vi "Main.vi"() -> ()   [LabVIEW 2014]
uses:
  Lib/Formula/EnumFormula.ctl
  <vilib>/Utility/miscctls.llb/LVRowAndColumnTypeDef.ctl
  <vilib>/Utility/file.llb/Read From Spreadsheet File (string).vi
  Lib/Formula/Formula(Table).vi
  Lib/Formula/Formula(Scalar).vi
  <vilib>/Utility/file.llb/Write To Spreadsheet File (string).vi
  GlobalData/GlobalData.vi
panel:
  in  "停止":bool
  in  "タブ制御器":T1(tab)
  in  "サンプリング周期(sec)":dbl=0.002 min=1e-05 format="%#.6f"
  in  "getCh":bool
  in  "rowChNum":i32=2
  in  "rowCutNum":i32
  in  "cutRow":bool
  in  "READ":bool
  in  "rowChPos":i32=2 caption="CH名称範囲"
  in  "rowCutPos":i32 caption="ヘッダ部削除範囲"
  in  "入力データファイル":path
  in  "colCutNum":i32=2
  in  "cutCol":bool
  in  "colCutPos":i32=9 caption="不要列削除範囲"
  in  "Waveグラフ表示":bool
  in  "XYグラフ表示":bool
  in  "X軸列(1～)":i32=2
  in  "直接数値入力する":bool
  in  "B2値":dbl
  in  "追加となるCH名称":string
  in  "列追加":bool
  in  "B値":u16(ring) items=["No.", "時間HH:MM:SS.S", "M1回転rpm", "M2回転rpm", "M3回転rpm", "M1トルクN･m", "M2トルクN･m", "M3トルクN･m", "", "", "", "", "", "", "", "", "", "", "供試体温度1℃", "供試体温度2℃", "供試体温度3℃", "動力盤温度℃", "軸受温度1℃", "軸受温度2℃", "軸受温度3℃", "", "効率"]
  in  "式":T2
  in  "A値":u16(ring) items=["No.", "時間HH:MM:SS.S", "M1回転rpm", "M2回転rpm", "M3回転rpm", "M1トルクN･m", "M2トルクN･m", "M3トルクN･m", "", "", "", "", "", "", "", "", "", "", "供試体温度1℃", "供試体温度2℃", "供試体温度3℃", "動力盤温度℃", "軸受温度1℃", "軸受温度2℃", "軸受温度3℃", "", "効率"]
  in  "WRITE":bool
  in  "出力ファイル名":path
  in  "出力ファイル名（TDMS形式）":path
  in  "TDMSViewer":bool
  in  "TDMSで保存":bool
  in  "操作（0:open）":T3(ring)=enum."create or replace"
  in  "グループ名":string
  in  "新グラフ":bool
  in  "Nixedグラフ表示":bool
  in  "GraphViewer":bool
  in  "表":string[][](table)
  # "~"
  # "~"
  # "行"
  # "~"
  # "列"
  # "行"
  # "列を追加する"
  # "＝"
  # "テキスト形式でファイル保存"
  # "複数の波形データを１つのTDMSファイル形式にまとめる事が可能。"
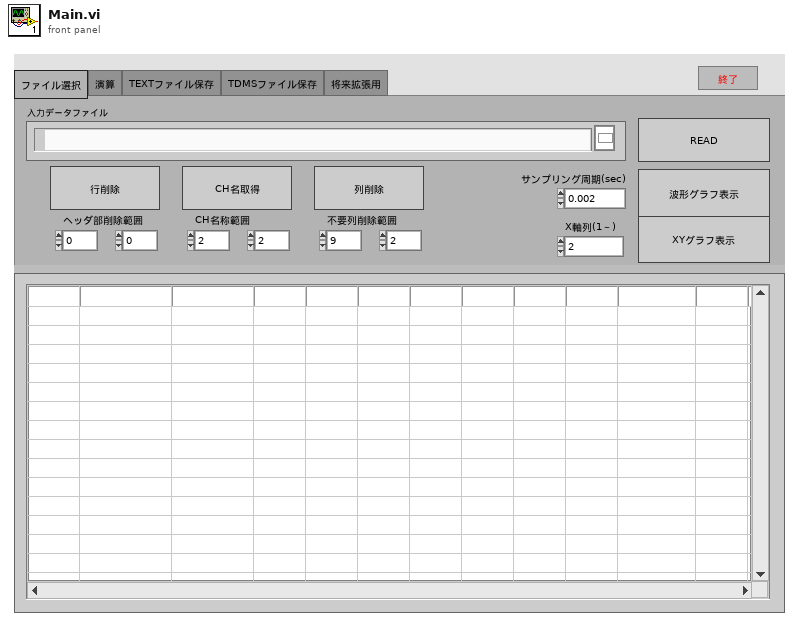
[diagram p1: front panel]
types:
  T1 = enum32{"ファイル選択", "演算", "TEXTファイル保存", "TDMSファイル保存", "将来拡張用"}
  T2 = typedef "EnumFormula.ctl" = enum16{"＋", "－", "×"}
  T3 = enum16{"open", "open or create", "create or replace", "create", "open (read-only)"}
  T4 = enum8{"Enabled", "Disabled", "Disabled and Grayed Out"}
  T5 = typedef "LVRowAndColumnTypeDef.ctl" = cluster{"Row":i32, "Column":i32}
  T6 = enum32{"Invalid", "Standard", "Closed", "Hidden", "Minimized", "Maximized"}
  T7 = typedef "LVRowAndColumnUnsignedTypeDef.ctl" = cluster{"Row":u32, "Column":u32}
  T8 = typedef "BoolSignalChangeCheck.ctl" = enum16{"OFF中", "立上り", "立下り", "ON中"}
  T9 = enum32{"Bad", "Idle", "Run top level", "Running"}
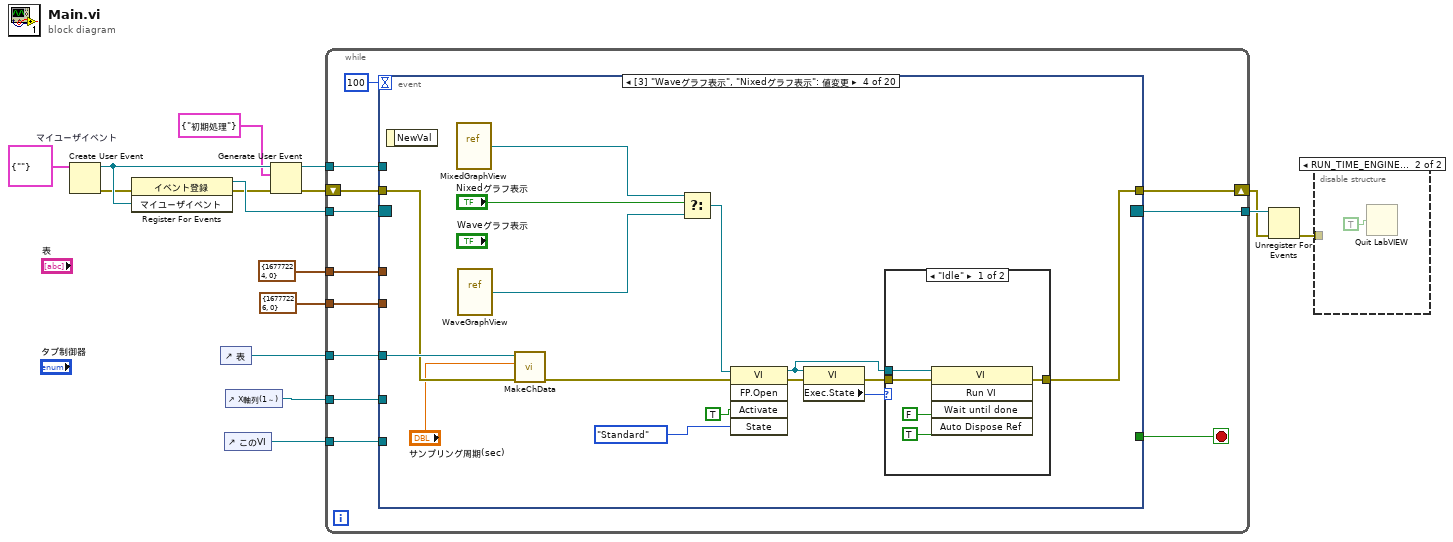
[diagram p0: block diagram]
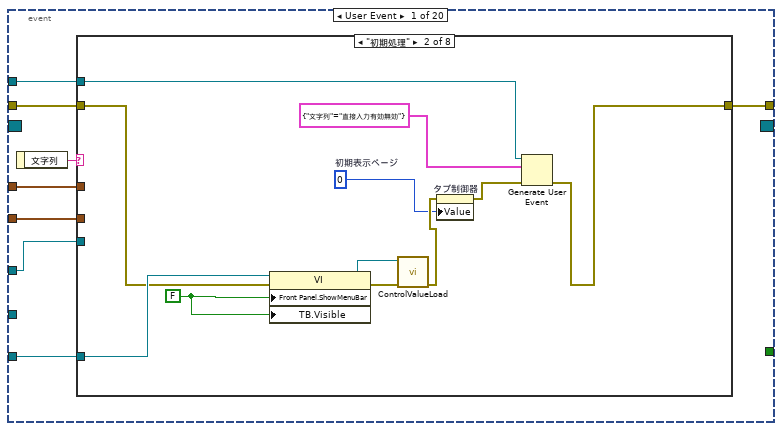
[diagram p3: hidden frame]
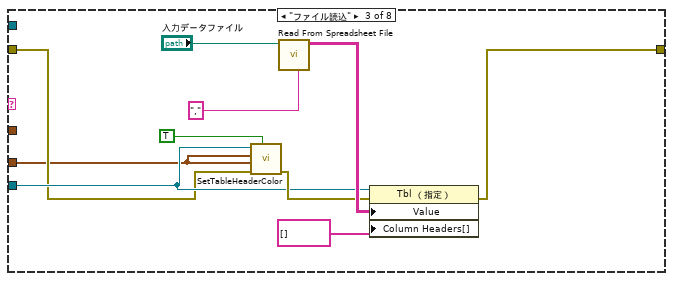
[diagram p5: hidden frame]
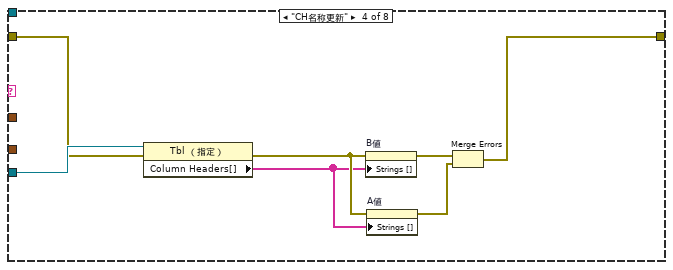
[diagram p6: hidden frame]
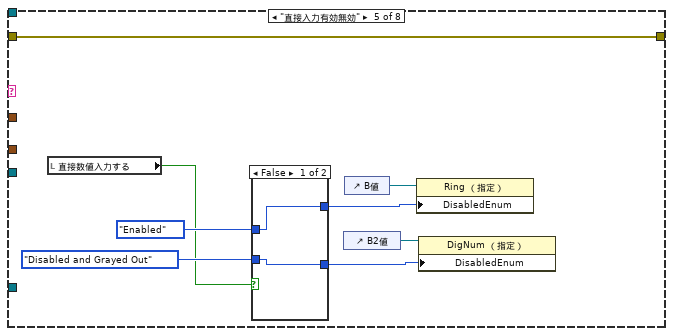
[diagram p7: hidden frame]
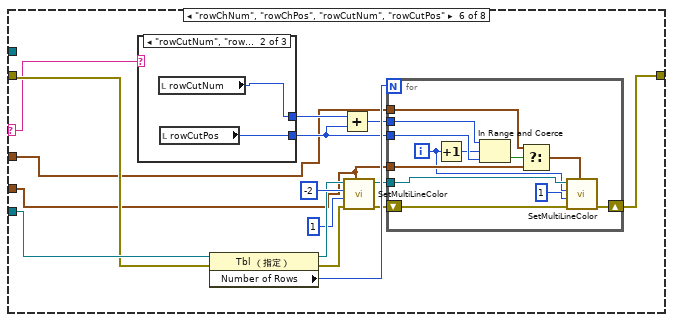
[diagram p9: hidden frame]
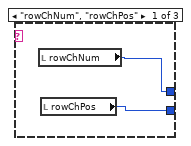
[diagram p10: hidden frame]
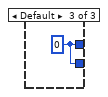
[diagram p11: hidden frame]
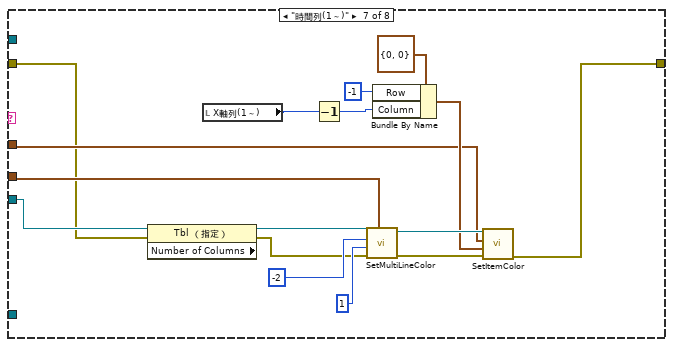
[diagram p12: hidden frame]
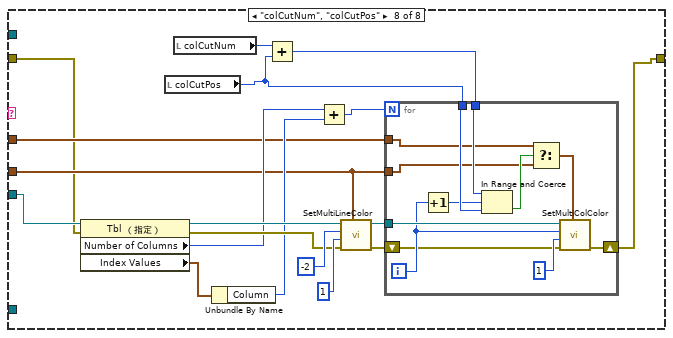
[diagram p13: hidden frame]
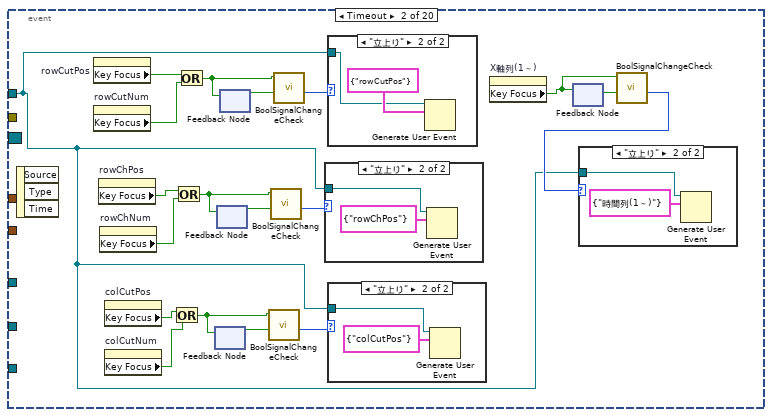
[diagram p14: hidden frame]
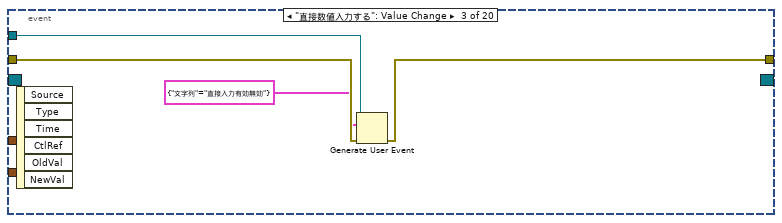
[diagram p19: hidden frame]
diagram:
  w12 = cluster{"文字列":string} {"文字列"=""}  # マイユーザイベント
  n1 = Create User Event(user event datatype=w12) -> (user event=w14:refnum<user-event>, error out=w5:errorcluster)  [unwired: 1 in]
  n2 = register-events(error in=w5, w14) -> (reference out=w16:refnum<event-registration>, error out=w4:errorcluster)  [unwired: 1 in]
  n3 = control-ref of="表"() -> (w10:refnum<vi>)
  n4 = control-ref of="このVI"() -> (w6:refnum<vi>)
  n5 = control-ref of="X軸列(1～)"() -> (w7:refnum<vi>)
  n6 = Generate User Event(user event=w14, event data cluster=cluster{"文字列":string} {"文字列"="初期処理"} ("イベントデータ"), error in=w4) -> (user event out=w13:refnum<user-event>, error out=w3:errorcluster)  [unwired: 1 in]
  n7 = while {
    tunnel: w16 -> [w27]
    tunnel: w13 -> [w26]
    tunnel: [w25] -> w15
    tunnel: w10 -> [w24]
    tunnel: cluster{"背景色":u32, "文字色":u32} {"背景色"=16777226, "文字色"=0} ("色指定") -> [w23]
    tunnel: cluster{"背景色":u32, "文字色":u32} {"背景色"=16777224, "文字色"=0} ("色指定") -> [w22]
    tunnel: w7 -> [w21]
    tunnel: w6 -> [w20]
    shift-right: [w18] -> w1
    shift-left: w3 -> [w19]
    stop <- w28 stop-if-true
    n8 = event shown="[3] \"Waveグラフ表示\", \"Nixedグラフ表示\": 値変更" {
      selector: w27 -> [_ _ _ _ _ _ _ _ _ _ _ _ _ _ _ _ _ _ _ _]
      dyn-events: [_ _ _ _ _ _ _ _ _ _ _ _ _ _ _ _ _ _ _ _] -> w25
      timeout: 100 -> [_ _ _ _ _ _ _ _ _ _ _ _ _ _ _ _ _ _ _ _]
      tunnel: [_ _ _ _ _ _ _ _ _ _ _ _ _ _ _ _ _ _ _ "停止"] -> w28
      tunnel: w26 -> [w35 w157 w184 _ _ _ w235 _ _ _ _ w315 w319 w323 w335 w336 _ w361 w386 _]
      tunnel: w24 -> [w34 _ _ w192 w211 w218 w232 w258 _ w278 w300 _ _ _ _ _ w343 w376 w383 w412]
      tunnel: w23 -> [w30 _ _ _ _ _ _ _ _ _ _ _ _ _ _ _ w356 w370 w389 w410]
      tunnel: w22 -> [w29 _ _ _ _ _ _ _ _ _ _ _ _ _ _ _ _ _ _ _]
      tunnel: w21 -> [_ _ _ _ _ w219 _ _ _ _ _ _ _ _ _ _ _ _ _ _]
      tunnel: w20 -> [w33 _ _ _ _ _ _ _ _ _ _ _ _ _ _ _ _ _ _ w403]
      tunnel: w19 -> [w32 _ w187 w191 w213 w217 w226 w255 w271 w277 w298 w316 w318 w327 w334 w342 w344 w358 w385 w406]
      tunnel: [w31 _ w186 w189 w212 w215 w223 w253 w270 _ w297 w313 w317 w321 w333 w341 w345 w359 w384 w400] -> w18
      event User Event {
        n9 = event-data() -> ("文字列"=w36:string)  [unwired: 1 in]
        n10 = case shown="\"初期処理\"" w36 {
          selector: w36 -> [_ _ _ _ _ w81 _ _]
          tunnel: w35 -> [_ w42 _ _ _ _ _ _]
          tunnel: w34 -> [_ _ w52 w65 _ w83 w113 w129]
          tunnel: w33 -> [_ w47 _ _ _ _ _ _]
          tunnel: w32 -> [w37 w45 w51 w64 w67 w82 w112 w127]
          tunnel: [w37 w41 w50 w60 w67 w80 w111 w128] -> w31
          tunnel: w30 -> [_ _ w49 _ _ w78 w114 w130]
          tunnel: w29 -> [_ _ _ _ _ w79 w115 w131]
          frame Default {
          }
          frame "初期処理" {
            w38 = u32 0  # 初期表示ページ
            w48 = FALSE
            n11 = property class="VI"(reference=w47, error in=w45, "Front Panel.ShowMenuBar"=w48, "TB.Visible"=w48) -> (reference out=w46:refnum<vi>, error out=w44:errorcluster)
            n12 = call "ControlValueLoad.vi"("err(in)"=w44, "VI refnum"=w46) -> ("err(out)"=w39:errorcluster)  [unwired: 9 in]
            n13 = property on="タブ制御器" class="TabCtl （指定）"(error in=w39, "Value"=w38) -> (error out=w40:errorcluster)  [unwired: 1 in, 1 out]
            n14 = Generate User Event(user event=w42, event data cluster=cluster{"文字列":string} {"文字列"="直接入力有効無効"} ("イベントデータ"), error in=w40) -> (error out=w41:errorcluster)  [unwired: 1 in, 1 out]
          }
          frame "ファイル読込" {
            n15 = call "SetTableHeaderColor.vi"("セル塗?(F)"=TRUE, "エラー入力(エラーなし)"=w51, "セル色指定"=w49, "ヘッダー色指定"=w49, "Tbl refnum"=w52) -> ("エラー出力"=w53:errorcluster)  [unwired: 6 in]
            n16 = call-poly <vilib>:"Read From Spreadsheet File.vi"("delimiter (\\t)"="," ("delimiter (\\t)"), "file path (dialog if empty)"="入力データファイル") -> ("all rows"=w55:string[][])  [unwired: 5 in, 4 out]
            n17 = property class="Tbl （指定）"(reference=w52, error in=w53, "Value"=w55, "Column Headers[]"=string[] [] ("行ヘッダ文字列[]")) -> (error out=w50:errorcluster)  [unwired: 1 out]
          }
          frame "CH名称更新" {
            n18 = property class="Tbl （指定）"(reference=w65, error in=w64) -> (error out=w63:errorcluster, "Column Headers[]"=w59:string[])  [unwired: 1 out]
            n19 = property on="B値" class="Ring （指定）"(error in=w63, "Strings []"=w59) -> (error out=w62:errorcluster)  [unwired: 1 in, 1 out]
            n20 = property on="A値" class="Ring （指定）"(error in=w63, "Strings []"=w59) -> (error out=w61:errorcluster)  [unwired: 1 in, 1 out]
            n21 = Merge Errors(w62, w61) -> (w60:errorcluster)
          }
          frame "直接入力有効無効" {
            n22 = local read "直接数値入力する"() -> (w66:bool)
            n23 = case shown="FALSE" w66 {
              tunnel: [w75 w77] -> w71
              tunnel: T4."Enabled" ("無効") -> [w74 w77]
              tunnel: [w74 w76] -> w69
              tunnel: T4."Disabled and Grayed Out" ("無効") -> [w75 w76]
              frame False {
              }
              frame True {
              }
            }
            n24 = control-ref of="B2値"() -> (w72:refnum<vi>)
            n25 = control-ref of="B値"() -> (w73:refnum<vi>)
            n26 = property class="Ring （指定）"(reference=w73, "DisabledEnum"=w69) -> ()  [unwired: 1 in, 2 out]
            n27 = property class="DigNum （指定）"(reference=w72, "DisabledEnum"=w71) -> ()  [unwired: 1 in, 2 out]
          }
          frame "rowChNum", "rowChPos", "rowCutNum", "rowCutPos" {
            n28 = case shown="\"rowCutNum\", \"rowCutPos\"" w81 {
              tunnel: [w95 w97 w98] -> w90
              tunnel: [w94 w96 w98] -> w92
              frame "rowChNum", "rowChPos" {
                n29 = local read "rowChNum"() -> (w95:i32)
                n30 = local read "rowChPos"() -> (w94:i32)
              }
              frame "rowCutNum", "rowCutPos" {
                n31 = local read "rowCutNum"() -> (w97:i32)
                n32 = local read "rowCutPos"() -> (w96:i32)
              }
              frame Default {
                w98 = 0
              }
            }
            n33 = property class="Tbl （指定）"(reference=w83, error in=w82) -> (reference out=w87:refnum<vi>, error out=w85:errorcluster, "Number of Rows"=w93:u32)
            n34 = Add(x=w90, y=w92) -> (x+y=w91:i32)
            n35 = call "SetMultiLineColor.vi"("色指定"=w78, "Error In"=w85, "長さ"=1, "開始行"=-2, "Tbl refnum"=w87) -> ("Error Out"=w84:errorcluster, "Tbl refnum出力"=w88:refnum<vi>)  [unwired: 5 in]
            n36 = for {
              N: w93 -> [_]
              tunnel: w91 -> [w110]
              tunnel: w92 -> [w109]
              tunnel: w79 -> [w107]
              tunnel: w78 -> [w106]
              tunnel: w88 -> [w104]
              shift-right: [w99] -> w80
              shift-left: w84 -> [w100]
              i -> [w103]
              n37 = Increment(x=w103) -> (x+1=w101:i32)
              n38 = In Range and Coerce(upper limit=w110, x=w101, lower limit=w109) -> (In Range?=w108:bool)  [unwired: 1 out]
              n39 = Select(t=w107, s=w108, f=w106) -> (s? t:f=w105:cluster{"背景色":u32, "文字色":u32})
              n40 = call "SetMultiLineColor.vi"("色指定"=w105, "Error In"=w100, "長さ"=1, "開始行"=w103, "Tbl refnum"=w104) -> ("Error Out"=w99:errorcluster)  [unwired: 5 in, 1 out]
            }
          }
          frame "時間列(1～)" {
            n41 = property class="Tbl （指定）" props=["Number of Columns"](reference=w113, error in=w112) -> (reference out=w126:refnum<vi>, error out=w123:errorcluster)  [unwired: 1 out]
            n42 = local read "X軸列(1～)"() -> (w116:i32)
            n43 = Decrement(x=w116) -> (x-1=w117:i32)
            n44 = call "SetMultiLineColor.vi"("色指定"=w114, "Error In"=w123, "長さ"=1, "開始行"=-2, "Tbl refnum"=w126) -> ("Error Out"=w119:errorcluster, "Tbl refnum出力"=w120:refnum<vi>)  [unwired: 5 in]
            n45 = Bundle By Name(cluster=T5 {"Row"=0, "Column"=0} ("行列指定"), "Row"=-1, "Column"=w117) -> (w118:T5)
            n46 = call "SetItemColor.vi"("エラー入力(エラーなし)"=w119, "行列指定"=w118, "色指定"=w115, "Tbl refnum"=w120) -> ("エラー出力"=w111:errorcluster)  [unwired: 7 in]
          }
          frame "colCutNum", "colCutPos" {
            n47 = property class="Tbl （指定）"(reference=w129, error in=w127) -> (reference out=w142:refnum<vi>, error out=w139:errorcluster, "Number of Columns"=w135:u32, "Index Values"=w137:T7)
            n48 = local read "colCutPos"() -> (w132:i32)
            n49 = local read "colCutNum"() -> (w133:i32)
            n50 = Unbundle By Name(w137) -> ("Column"=w136:u32)
            n51 = Add(x=w133, y=w132) -> (x+y=w144:i32)
            n52 = Add(x=w135, y=w136) -> (x+y=w134:u32)
            n53 = call "SetMultiLineColor.vi"("色指定"=w130, "Error In"=w139, "長さ"=1, "開始行"=-2, "Tbl refnum"=w142) -> ("Error Out"=w138:errorcluster, "Tbl refnum出力"=w141:refnum<vi>)  [unwired: 5 in]
            n54 = for {
              N: w134 -> [_]
              tunnel: w144 -> [w156]
              tunnel: w132 -> [w155]
              tunnel: w131 -> [w153]
              tunnel: w130 -> [w152]
              tunnel: w141 -> [w150]
              shift-right: [w145] -> w128
              shift-left: w138 -> [w146]
              i -> [w149]
              n55 = Increment(x=w149) -> (x+1=w147:i32)
              n56 = In Range and Coerce(upper limit=w156, x=w147, lower limit=w155) -> (In Range?=w154:bool)  [unwired: 1 out]
              n57 = Select(t=w153, s=w154, f=w152) -> (s? t:f=w151:cluster{"背景色":u32, "文字色":u32})
              n58 = call "SetMultiColColor.vi"("色指定"=w151, "Error In"=w146, "長さ"=1, "開始列"=w149, "Tbl refnum"=w150) -> ("Error Out"=w145:errorcluster)  [unwired: 5 in, 1 out]
            }
          }
        }
      }
      event Timeout {
        n59 = event-data() -> ()  [unwired: 1 in, 3 out]
        n60 = property on="rowCutPos" class="DigNum （指定）"() -> ("Key Focus"=w175:bool)  [unwired: 2 in, 2 out]
        n61 = property on="rowCutNum" class="DigNum （指定）"() -> ("Key Focus"=w174:bool)  [unwired: 2 in, 2 out]
        n62 = property on="rowChPos" class="DigNum （指定）"() -> ("Key Focus"=w167:bool)  [unwired: 2 in, 2 out]
        n63 = property on="rowChNum" class="DigNum （指定）"() -> ("Key Focus"=w166:bool)  [unwired: 2 in, 2 out]
        n64 = property on="colCutPos" class="DigNum （指定）"() -> ("Key Focus"=w163:bool)  [unwired: 2 in, 2 out]
        n65 = property on="colCutNum" class="DigNum （指定）"() -> ("Key Focus"=w162:bool)  [unwired: 2 in, 2 out]
        n66 = Or(x=w163, y=w162) -> (x .or. y?=w165:bool)
        n67 = Or(x=w167, y=w166) -> (x .or. y?=w168:bool)
        n68 = Or(x=w175, y=w174) -> (x .or. y?=w173:bool)
        n69 = feedback #1() -> (w164:bool)  [unwired: 1 in]
        n70 = feedback-in #1(w165) -> ()
        n71 = feedback #2() -> (w169:bool)  [unwired: 1 in]
        n72 = feedback-in #2(w168) -> ()
        n73 = feedback-in #3(w173) -> ()
        n74 = feedback #3() -> (w172:bool)  [unwired: 1 in]
        n75 = call "BoolSignalChangeCheck.vi"("前回値"=w164, "今回値"=w165) -> ("判定"=w161:T8)  [unwired: 9 in]
        n76 = call "BoolSignalChangeCheck.vi"("前回値"=w169, "今回値"=w168) -> ("判定"=w170:T8)  [unwired: 9 in]
        n77 = call "BoolSignalChangeCheck.vi"("前回値"=w172, "今回値"=w173) -> ("判定"=w171:T8)  [unwired: 9 in]
        n78 = case shown="\"立上り\"" w170 {
          tunnel: w157 -> [_ w180]
          frame "OFF中", Default {
          }
          frame "立上り" {
            n79 = Generate User Event(user event=w180, event data cluster=cluster{"文字列":string} {"文字列"="rowChPos"} ("イベントデータ")) -> ()  [unwired: 2 in, 2 out]
          }
        }
        n80 = case shown="\"立上り\"" w171 {
          tunnel: w157 -> [_ w182]
          frame "OFF中", Default {
          }
          frame "立上り" {
            n81 = Generate User Event(user event=w182, event data cluster=cluster{"文字列":string} {"文字列"="rowCutPos"} ("イベントデータ")) -> ()  [unwired: 2 in, 2 out]
          }
        }
        n82 = case shown="\"立上り\"" w161 {
          tunnel: w157 -> [_ w178]
          frame "OFF中", Default {
          }
          frame "立上り" {
            n83 = Generate User Event(user event=w178, event data cluster=cluster{"文字列":string} {"文字列"="colCutPos"} ("イベントデータ")) -> ()  [unwired: 2 in, 2 out]
          }
        }
        n84 = property on="X軸列(1～)" class="DigNum （指定）"() -> ("Key Focus"=w160:bool)  [unwired: 2 in, 2 out]
        n85 = feedback #4() -> (w159:bool)  [unwired: 1 in]
        n86 = feedback-in #4(w160) -> ()
        n87 = call "BoolSignalChangeCheck.vi"("前回値"=w159, "今回値"=w160) -> ("判定"=w158:T8)  [unwired: 9 in]
        n88 = case shown="\"立上り\"" w158 {
          tunnel: w157 -> [_ w176]
          frame "OFF中", Default {
          }
          frame "立上り" {
            n89 = Generate User Event(user event=w176, event data cluster=cluster{"文字列":string} {"文字列"="時間列(1～)"} ("イベントデータ")) -> ()  [unwired: 2 in, 2 out]
          }
        }
      }
      event "直接数値入力する": Value Change {
        n90 = event-data() -> ()  [unwired: 1 in, 6 out]
        n91 = Generate User Event(user event=w184, event data cluster=cluster{"文字列":string} {"文字列"="直接入力有効無効"} ("イベントデータ"), error in=w187) -> (error out=w186:errorcluster)  [unwired: 1 in, 1 out]
      }
      event "Waveグラフ表示", "Nixedグラフ表示": Value Change {
        n92 = event-data() -> ()  [unwired: 1 in, 1 out]
        n93 = vi-ref "MixedGraphView.vi"() -> (w196:refnum<vi>)
        n94 = vi-ref "WaveGraphView.vi"() -> (w195:refnum<vi>)
        n95 = call "MakeChData.vi"("error in (no error)"=w191, "サンプリング周期(sec)"="サンプリング周期(sec)", "表 ref"=w192) -> ("error out"=w193:errorcluster)  [unwired: 8 in]
        n96 = Select(t=w196, s="Nixedグラフ表示", f=w195) -> (s? t:f=w194:refnum<vi>)
        n97 = invoke class="VI" method="FP.Open"(reference=w194, error in=w193, "Activate"=TRUE ("アクティブ化?"), "State"=T6."Standard" ("状態")) -> (reference out=w200:refnum<vi>, error out=w199:errorcluster)  [unwired: 1 in, 3 out]
        n98 = property class="VI"(reference=w200, error in=w199) -> (error out=w190:errorcluster, "Exec.State"=w198:T9)  [unwired: 1 out]
        n99 = case shown="\"Idle\"" w198 {
          tunnel: w200 -> [w205 _]
          tunnel: w190 -> [w204 w208]
          tunnel: [w203 w208] -> w189
          frame "Idle" {
            n100 = invoke class="VI" method="Run VI"(reference=w205, error in=w204, "Wait until done"=FALSE ("終了まで待機"), "Auto Dispose Ref"=TRUE ("リファレンスを自動破棄")) -> (error out=w203:errorcluster)  [unwired: 1 in, 4 out]
          }
          frame Default {
          }
        }
      }
      event "新グラフ": Value Change {
        n101 = event-data() -> ()  [unwired: 1 in, 1 out]
        n102 = vi-ref "GraphView.vi"() -> (w210:refnum<vi>)
        n103 = local read "サンプリング周期(sec)"() -> (w209:dbl)
        n104 = call "MakeChData.vi"("error in (no error)"=w213, "サンプリング周期(sec)"=w209, "表 ref"=w211) -> ("error out"=w214:errorcluster)  [unwired: 8 in]
        n105 = call "FormPopup.vi"("エラー入力（エラーなし）"=w214, "VI入力"=w210) -> ("エラー出力"=w212:errorcluster)  [unwired: 9 in]
      }
      event "XYグラフ表示": Value Change {
        n106 = event-data() -> ()  [unwired: 1 in, 1 out]
        n107 = call "MakeXyData.vi"("error in (no error)"=w217, "時間列(1～) ref"=w219, "表 ref"=w218) -> ("error out"=w216:errorcluster)  [unwired: 8 in]
        n108 = vi-ref "XYGraphView.vi"() -> (w220:refnum<vi>)
        n109 = call "FormPopup.vi"("エラー入力（エラーなし）"=w216, "VI入力"=w220) -> ("エラー出力"=w215:errorcluster)  [unwired: 9 in]
      }
      event "列追加": Value Change {
        n110 = event-data() -> ()  [unwired: 1 in, 1 out]
        n111 = property class="Tbl （指定）"(reference=w232, error in=w226) -> (reference out=w230:refnum<vi>, error out=w225:errorcluster, "Value"=w222:string[][])
        n112 = Transpose 2D Array(2D array=w222) -> (transposed array=w221:string[][])
        n113 = case shown="TRUE" "直接数値入力する" {
          tunnel: "A値" -> [w244 w250]
          tunnel: "B値" -> [w243 _]
          tunnel: [w241 w252] -> w236
          tunnel: "B2値" -> [_ w249]
          tunnel: "式" -> [w242 w248]
          tunnel: w221 -> [w245 w251]
          tunnel: w225 -> [w240 w247]
          tunnel: [w239 w246] -> w224
          frame False {
            n114 = call-poly "Formula.vi"("式"=w242, "error in (no error)"=w240, "B値(列位置 0～)"=w243, "A値(列位置 0～)"=w244, "元データ(2D)"=w245) -> ("error out"=w239:errorcluster, "結果データ(1D)"=w241:dbl[])  [unwired: 5 in]
          }
          frame True {
            n115 = call-poly "Formula.vi"("式"=w248, "error in (no error)"=w247, "B(値)"=w249, "A(列位置 0～)"=w250, "元データ(2D)"=w251) -> ("error out"=w246:errorcluster, "結果データ(1D)"=w252:dbl[])  [unwired: 5 in]
          }
        }
        n116 = call "AddColData.vi"("エラー入力（エラーなし）"=w224, "名称"="追加となるCH名称", "配列"=w236, "Table入力"=w230) -> ("エラー出力"=w231:errorcluster)  [unwired: 7 in]
        n117 = Generate User Event(user event=w235, event data cluster=cluster{"文字列":string} {"文字列"="Ch名称更新"} ("イベントデータ"), error in=w231) -> (error out=w223:errorcluster)  [unwired: 1 in, 1 out]
      }
      event "WRITE": Value Change {
        n118 = event-data() -> ()  [unwired: 1 in, 1 out]
        n119 = property class="Tbl （指定）"(reference=w258, error in=w255) -> (error out=w254:errorcluster, "Column Headers[]"=w257:string[], "Value"=w256:string[][])  [unwired: 1 out]
        n120 = Build Array (concatenate)(w257, w256) -> (w259:string[][])
        n121 = call <vilib>:"Check if File or Folder Exists.vi"("error in (no error)"=w254, "path"="出力ファイル名") -> ("error out"=w253:errorcluster, "file or folder exists?"=w262:bool, "dup path"=w261:path)  [unwired: 7 in]
        n122 = case shown="TRUE" w262 {
          tunnel: [TRUE w268] -> w260
          frame False {
          }
          frame True {
            n123 = Two Button Dialog(message="上書きします。\n宜しいですか？" ("メッセージ")) -> (T button?=w268:bool)  [unwired: 2 in]
          }
        }
        n124 = case shown="TRUE" w260 {
          tunnel: w261 -> [_ w266]
          tunnel: w259 -> [_ w264]
          frame False {
          }
          frame True {
            n125 = call-poly <vilib>:"Write To Spreadsheet File.vi"("delimiter (\\t)"="," ("delimiter (\\t)"), "2D data"=w264, "file path (dialog if empty)"=w266) -> ()  [unwired: 5 in, 1 out]
          }
        }
      }
      event "TDMSViewer": Value Change {
        n126 = event-data() -> ()  [unwired: 1 in, 1 out]
        n127 = local read "出力ファイル名（TDMS形式）"() -> (w272:path)
        n128 = call <vilib>:"TDMS - File Viewer.vi"("error in (no error)"=w271, "file path"=w272) -> ("error out"=w270:errorcluster)  [unwired: 4 in, 1 out]
      }
      event "GraphViewer": Value Change {
        n129 = event-data() -> ()  [unwired: 1 in, 1 out]
        n130 = local read "サンプリング周期(sec)"() -> (w273:dbl)
        n131 = call "MakeChData.vi"("error in (no error)"=w277, "サンプリング周期(sec)"=w273, "表 ref"=w278) -> ("error out"=w276:errorcluster)  [unwired: 8 in]
        n132 = flat-sequence {
          tunnel: w276 -> [_]
          tunnel: [w283] -> w275
          tunnel: [w282] -> w274
          frame #0 {
            n133 = property on="入力データファイル" class="Path"() -> ("Text.Text"=w281:string)  [unwired: 2 in, 2 out]
            n134 = String To Path(string=w281) -> (path=w280:path)
            n135 = call <vilib>:"Application Directory.vi"() -> ("Application Directory"=w287:path)
            n136 = call <vilib>:"Get File Extension.vi"("file"=w280) -> ("filename without extension"=w279:string)  [unwired: 7 in, 3 out]
            n137 = Build Path(base path=w287, name or relative path="WaveDisp V2.tdms" ("名前または相対パス")) -> (appended path=w285:path)
            n138 = global read "GlobalData.vi" "ChName"() -> (w294:string[])
            n139 = global read "GlobalData.vi" "ChData"() -> (w293:waveform(dbl)[])
            n140 = TDMS Open(10:T3."create or replace" ("操作（0:open）"), 11:w285) -> (0:w292:errorcluster, 3:w295:refnum<k34>)  [unwired: 5 in]
            n141 = TDMS Write(0:w295, 5:w279, 7:w294, 9:w293, 11:w292) -> (4:w290:refnum<k34>, 15:w291:errorcluster)  [unwired: 1 in, 2 out]
            n142 = TDMS Flush(4:w291, 7:w290) -> (0:w289:errorcluster, 3:w288:refnum<k34>)
            n143 = TDMS Close(8:w289, 11:w288) -> (0:w283:errorcluster, 3:w282:path)
          }
        }
        n144 = call <vilib>:"TDMS - File Viewer.vi"("error in (no error)"=w275, "file path"=w274) -> ()  [unwired: 4 in, 2 out]
      }
      event "TDMSで保存": Value Change {
        n145 = event-data() -> ()  [unwired: 1 in, 1 out]
        n146 = local read "サンプリング周期(sec)"() -> (w296:dbl)
        n147 = call "MakeChData.vi"("error in (no error)"=w298, "サンプリング周期(sec)"=w296, "表 ref"=w300) -> ("error out"=w299:errorcluster)  [unwired: 8 in]
        n148 = flat-sequence {
          tunnel: w299 -> [w301]
          tunnel: [w301] -> w297
          frame #0 {
            n149 = global read "GlobalData.vi" "ChName"() -> (w308:string[])
            n150 = global read "GlobalData.vi" "ChData"() -> (w307:waveform(dbl)[])
            n151 = TDMS Open(10:"操作（0:open）", 11:"出力ファイル名（TDMS形式）") -> (0:w306:errorcluster, 3:w312:refnum<k34>)  [unwired: 5 in]
            n152 = TDMS Write(0:w312, 5:"グループ名", 7:w308, 9:w307, 11:w306) -> (4:w304:refnum<k34>, 15:w305:errorcluster)  [unwired: 1 in, 2 out]
            n153 = TDMS Flush(4:w305, 7:w304) -> (0:w303:errorcluster, 3:w302:refnum<k34>)
            n154 = TDMS Close(8:w303, 11:w302) -> ()  [unwired: 2 out]
          }
        }
      }
      event "READ": Value Change {
        n155 = event-data() -> ()  [unwired: 1 in, 1 out]
        n156 = Generate User Event(user event=w315, event data cluster=cluster{"文字列":string} {"文字列"="ファイル読込"} ("イベントデータ"), error in=w316) -> (error out=w313:errorcluster)  [unwired: 1 in, 1 out]
      }
      event "入力データファイル": Value Change {
        n157 = event-data() -> ()  [unwired: 1 in, 1 out]
        n158 = Generate User Event(user event=w319, event data cluster=cluster{"文字列":string} {"文字列"="ファイル読込"} ("イベントデータ"), error in=w318) -> (error out=w317:errorcluster)  [unwired: 1 in, 1 out]
      }
      event "rowCutPos", "rowCutNum", "rowChNum", "rowChPos": Value Change {
        n159 = event-data() -> ("CtlRef"=w328:refnum<vi>)  [unwired: 1 in]
        n160 = property class="DigNum （指定）"(reference=w328, error in=w327) -> (error out=w322:errorcluster, "Label.Text"=w325:string)  [unwired: 1 out]
        n161 = Bundle By Name(cluster=cluster{"文字列":string} {"文字列"="(項目名)"} ("イベントデータ"), "文字列"=w325) -> (w324:cluster{"文字列":string})
        n162 = Generate User Event(user event=w323, event data cluster=w324, error in=w322) -> (error out=w321:errorcluster)  [unwired: 1 in, 1 out]
      }
      event "X軸列(1～)": Value Change {
        n163 = event-data() -> ("CtlRef"=w332:refnum<vi>)  [unwired: 1 in]
        n164 = property class="DigNum （指定）"(reference=w332) -> ("Label.Text"=w330:string)  [unwired: 1 in, 2 out]
        n165 = Bundle By Name(cluster=cluster{"文字列":string} {"文字列"="(項目名)"} ("イベントデータ"), "文字列"=w330) -> (w329:cluster{"文字列":string})
        n166 = Generate User Event(user event=w335, event data cluster=w329, error in=w334) -> (error out=w333:errorcluster)  [unwired: 1 in, 1 out]
      }
      event "colCutPos", "colCutNum": Value Change {
        n167 = event-data() -> ("CtlRef"=w340:refnum<vi>)  [unwired: 1 in]
        n168 = property class="DigNum （指定）"(reference=w340) -> ("Label.Text"=w338:string)  [unwired: 1 in, 2 out]
        n169 = Bundle By Name(cluster=cluster{"文字列":string} {"文字列"="(項目名)"} ("イベントデータ"), "文字列"=w338) -> (w337:cluster{"文字列":string})
        n170 = Generate User Event(user event=w336, event data cluster=w337, error in=w342) -> (error out=w341:errorcluster)  [unwired: 1 in, 1 out]
      }
      event "cutRow": Value Change {
        n171 = event-data() -> ()  [unwired: 1 in, 1 out]
        n172 = property class="Tbl （指定）"(reference=w343, error in=w344) -> (reference out=w351:refnum<vi>, error out=w350:errorcluster, "Value"=w357:string[][])
        n173 = local read "rowCutNum"() -> (w348:i32)
        n174 = local read "rowCutPos"() -> (w349:i32)
        n175 = Decrement(x=w349) -> (x-1=w346:i32)
        n176 = Delete From Array(array=w357, length=w348, index (row)=w346) -> (array with subset deleted=w347:string[][])  [unwired: 1 in, 1 out]
        n177 = property class="Tbl （指定）"(reference=w351, error in=w350, "Value"=w347) -> (reference out=w355:refnum<vi>, error out=w352:errorcluster, "Number of Rows"=w353:u32)
        n178 = call "SetMultiLineColor.vi"("色指定"=w356, "Error In"=w352, "長さ"=w353, "開始行"=-2, "Tbl refnum"=w355) -> ("Error Out"=w345:errorcluster)  [unwired: 5 in, 1 out]
      }
      event "getCh": Value Change {
        n179 = event-data() -> ()  [unwired: 1 in, 1 out]
        n180 = property class="Tbl （指定）"(reference=w376, error in=w358) -> (reference out=w371:refnum<vi>, error out=w363:errorcluster, "Value"=w375:string[][])
        n181 = local read "rowChNum"() -> (w368:i32)
        n182 = local read "rowChPos"() -> (w377:i32)
        n183 = Decrement(x=w377) -> (x-1=w367:i32)
        n184 = Delete From Array(array=w375, length=w368, index (row)=w367) -> (deleted portion=w366:string[][], array with subset deleted=w369:string[][])  [unwired: 1 in]
        n185 = call "MakeColHeaderString.vi"("CH名称(複数行)"=w366) -> ("CH名称(1行)"=w364:string[])  [unwired: 10 in]
        n186 = property class="Tbl （指定）"(reference=w371, error in=w363, "Value"=w369, "Column Headers[]"=w364) -> (reference out=w374:refnum<vi>, error out=w372:errorcluster, "Number of Rows"=w365:u32)
        n187 = call "SetMultiLineColor.vi"("色指定"=w370, "Error In"=w372, "長さ"=w365, "開始行"=-2, "Tbl refnum"=w374) -> ("Error Out"=w360:errorcluster)  [unwired: 5 in, 1 out]
        n188 = Generate User Event(user event=w361, event data cluster=cluster{"文字列":string} {"文字列"="CH名称更新"} ("イベントデータ"), error in=w360) -> (error out=w359:errorcluster)  [unwired: 1 in, 1 out]
      }
      event "cutCol": Value Change {
        n189 = event-data() -> ()  [unwired: 1 in, 1 out]
        n190 = property class="Tbl （指定）"(reference=w383, error in=w385) -> (reference out=w399:refnum<vi>, error out=w398:errorcluster, "Value"=w395:string[][], "Column Headers[]"=w381:string[])
        n191 = local read "colCutPos"() -> (w397:i32)
        n192 = local read "colCutNum"() -> (w378:i32)
        n193 = Decrement(x=w397) -> (x-1=w379:i32)
        n194 = Transpose 2D Array(2D array=w395) -> (transposed array=w394:string[][])
        n195 = Delete From Array(array=w394, length=w378, index (row)=w379) -> (array with subset deleted=w396:string[][])  [unwired: 1 in, 1 out]
        n196 = Delete From Array(array=w381, length=w378, index=w379) -> (array with subset deleted=w380:string[])  [unwired: 1 out]
        n197 = Transpose 2D Array(2D array=w396) -> (transposed array=w393:string[][])
        n198 = property class="Tbl （指定）"(reference=w399, error in=w398, "Value"=w393, "Column Headers[]"=w380) -> (reference out=w390:refnum<vi>, error out=w391:errorcluster, "Number of Columns"=w382:u32)
        n199 = call "SetMultiColColor.vi"("色指定"=w389, "Error In"=w391, "長さ"=w382, "開始列"=-2 ("開始行"), "Tbl refnum"=w390) -> ("Error Out"=w388:errorcluster)  [unwired: 5 in, 1 out]
        n200 = Generate User Event(user event=w386, event data cluster=cluster{"文字列":string} {"文字列"="CH名称更新"} ("イベントデータ"), error in=w388) -> (error out=w384:errorcluster)  [unwired: 1 in, 1 out]
      }
      event "停止": Value Change {
        w407 = TRUE
        n201 = event-data() -> ()  [unwired: 1 in, 1 out]
        n202 = property class="Tbl （指定）"(reference=w412, error in=w406, "Value"=string[][] [] ("値"), "Column Headers[]"=string[] [] ("列ヘッダ文字列[]")) -> (reference out=w409:refnum<vi>, error out=w405:errorcluster)
        n203 = call "SetMultiLineColor.vi"("色指定"=w410, "Error In"=w405, "長さ"=1, "開始行"=-2, "Tbl refnum"=w409) -> ("Error Out"=w404:errorcluster)  [unwired: 5 in, 1 out]
        n204 = property class="VI"(reference=w403, error in=w404, "TB.Visible"=w407, "Front Panel.ShowMenuBar"=w407) -> (reference out=w402:refnum<vi>, error out=w401:errorcluster)
        n205 = call "ControlValueSave.vi"("err(in)"=w401, "VI refnum"=w402) -> ("err(out)"=w400:errorcluster)  [unwired: 9 in]
      }
    }
  }
  n206 = Unregister For Events(event registration refnum=w15, error in=w1) -> (error out=w2:errorcluster)
  n207 = disable-structure shown="RUN_TIME_ENGINE==True" {
    disable-tunnel: w2 -> [_ _]
    frame condition #0 (active) {
    }
    frame condition #1 {
      n208 = Quit LabVIEW(quit? (T)=TRUE) -> ()
    }
  }
